vi "upload_data_db.vi"() -> ()   [LabVIEW 2021]
uses:
  <vilib>/Utility/file.llb/Read Delimited Spreadsheet (string).vi
panel:
  in  "function name 2":string="debugprint"
  out "Debug String Out":string="postgres"
  in  "Debug":bool
  out "String Out":string="Upload Success"
  in  "Data cluster":T1={"type"="proto", " geometry"="full", "resolution"="LD", "baselayer"="BA_123", "toplayer"="SI_789", "pos"="1", "region"="1", "asstray"="1", "comptray"="1", "put"="1", "date"="2024-04-02", "timestart"="1:12:12.442", "timeend"="1:23:45.244", "operator"="cmuperson", "tape"="some", "glue"="some"}
  out "Execution Time py":dbl=14.0
  in  "Python version":string="3.7.0"
  in  "stop":bool
  in  "Run Python":bool
  in  "function name":string="assembly_data"
  in  "module path":path=path "../../../Main VIs/python_db/postgres_tools.py"
  out "error out":errorcluster
  in  "error in (no error)":errorcluster
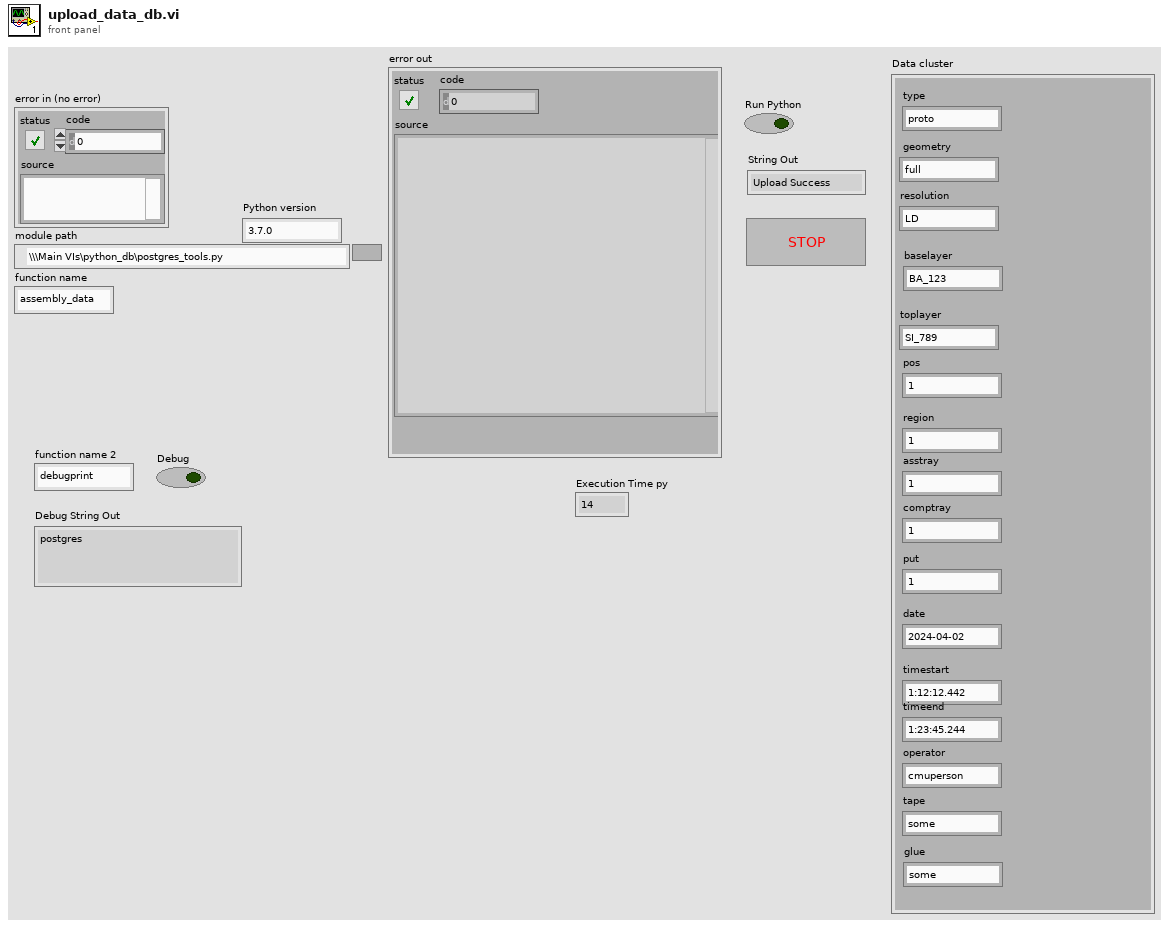
[diagram p1: front panel]
types:
  T1 = cluster{"type":string, " geometry":string, "resolution":string, "baselayer":string, "toplayer":string, "pos":string, "region":string, "asstray":string, "comptray":string, "put":string, "date":string, "timestart":string, "timeend":string, "operator":string, "tape":string, "glue":string}
  T2 = typedef "File Paths.ctl" = cluster{"Glue Pattern Folder":path, "Carrier Tray Folder":path, "Pick Up Tool Fixture Folder":path, "Components Folder":path, "Bellows Tool Offset.txt":path, "Pick Up Tool Offset.txt":path, "Dispense Tip Offset.txt":path, "Log Files":path, "Gantry Assembly Map.txt":path, "Syringe and offset map.txt":path, "Python DB Conn":path}
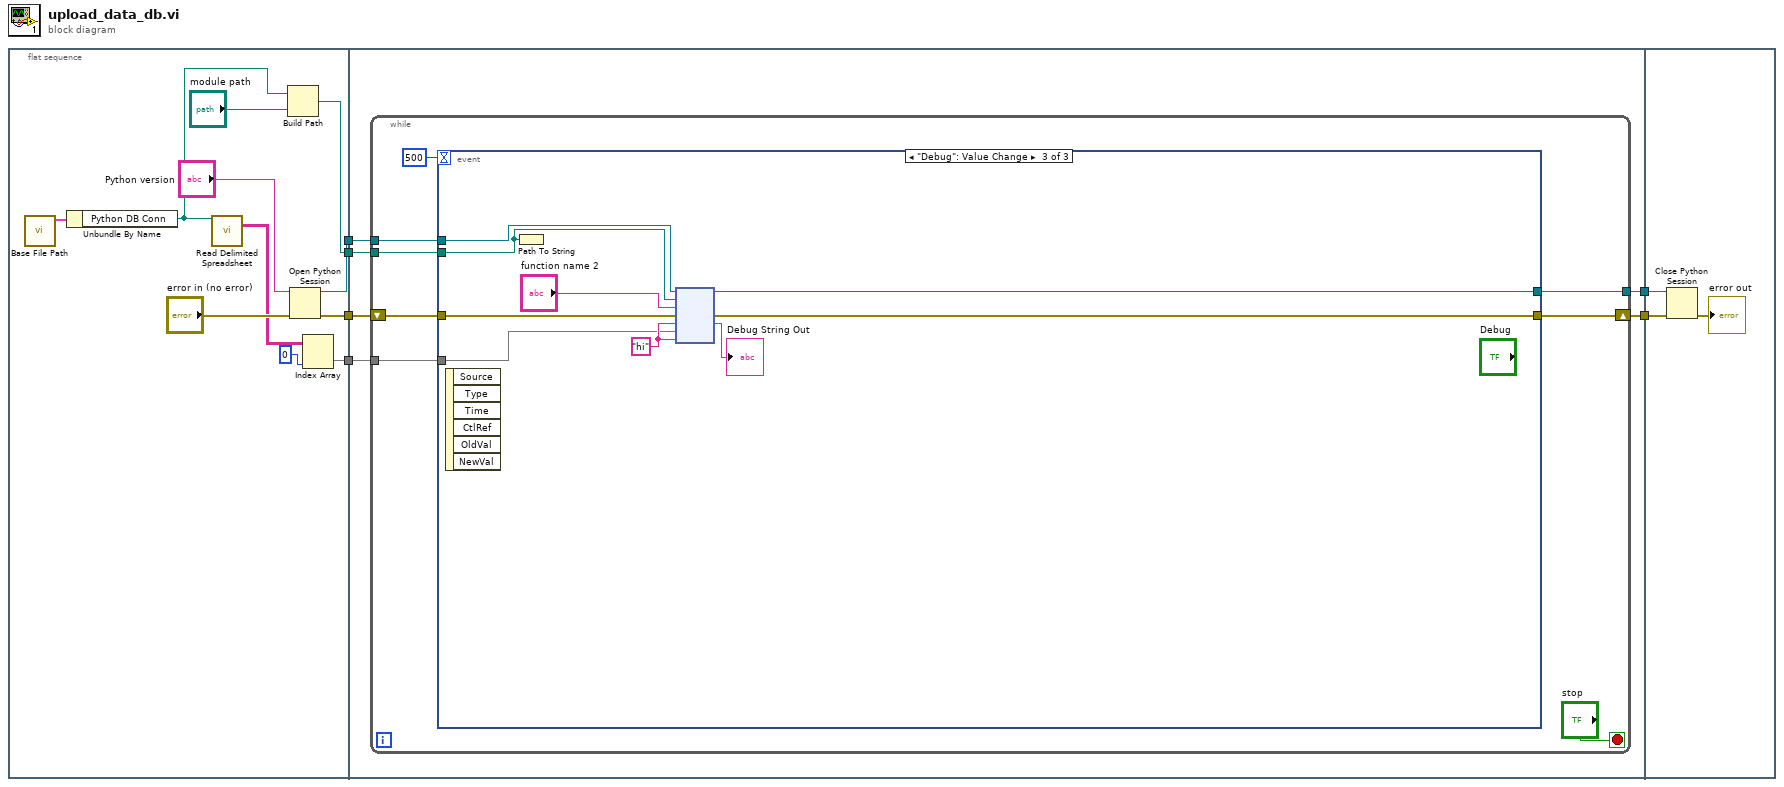
[diagram p0: block diagram]
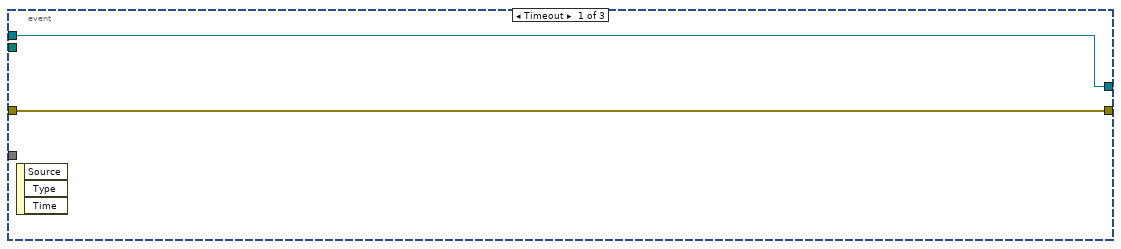
[diagram p2: hidden frame]
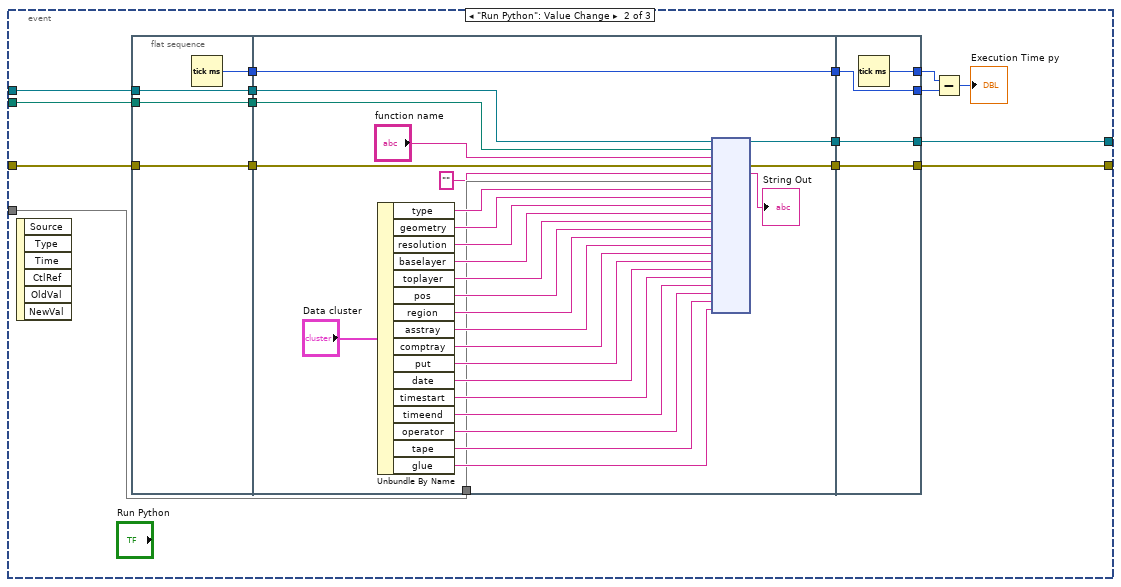
[diagram p3: hidden frame]
diagram:
  n1 = flat-sequence {
    tunnel: [w16] -> w4
    tunnel: [w17] -> w3
    tunnel: [w12] -> w2
    tunnel: [w7] -> w1
    tunnel: [w22] -> w6
    tunnel: [w21] -> w5
    tunnel: w4 -> [w23]
    tunnel: w3 -> [w20]
    tunnel: w2 -> [w19]
    tunnel: w1 -> [w18]
    tunnel: w6 -> [w95]
    tunnel: w5 -> [w96]
    frame #0 {
      n2 = call "Base File Path.vi"() -> ("Paths Out"=w13:T2)  [unwired: 11 in]
      n3 = Unbundle By Name(w13) -> ("Python DB Conn"=w10:path)
      n4 = call-poly <vilib>:"Read Delimited Spreadsheet.vi"("file path (dialog if empty)"=w10) -> ("all rows"=w9:string[][])  [unwired: 9 in, 5 out]
      n5 = Build Path(base path=w10, name or relative path="module path") -> (appended path=w12:path)
      n6 = Open Python Session(python version="Python version", 3:"error in (no error)") -> (session out=w17:refnum<k35>, error out=w16:errorcluster)  [unwired: 1 in]
      n7 = Index Array(array=w9, index (col)=0 ("disabled index (col)")) -> (element=w7:string[])  [unwired: 1 in]
    }
    frame #1 {
      n8 = while {
        shift-right: [w29] -> w22
        shift-left: w23 -> [w30]
        tunnel: w20 -> [w27]
        tunnel: [w28] -> w21
        tunnel: w19 -> [w25]
        tunnel: w18 -> [w24]
        stop <- "stop" stop-if-true
        n9 = event shown="[2] \"Debug\": Value Change" {
          selector: _ -> [_ _ _]
          dyn-events: _ -> [_ _ _]
          timeout: 500 -> [_ _ _]
          tunnel: [w33 w41 w92] -> w29
          tunnel: w30 -> [w33 w44 w93]
          tunnel: [w32 w39 w91] -> w28
          tunnel: w27 -> [w32 w38 w90]
          tunnel: w25 -> [_ w36 w88]
          tunnel: w24 -> [_ w34 w85]
          event Timeout {
            n10 = event-data() -> ()  [unwired: 1 in, 3 out]
          }
          event "Run Python": Value Change {
            n11 = event-data() -> ()  [unwired: 1 in, 6 out]
            n12 = flat-sequence {
              tunnel: [w53] -> w45
              tunnel: w44 -> [w52]
              tunnel: [w52] -> w43
              tunnel: w38 -> [w51]
              tunnel: [w51] -> w37
              tunnel: w36 -> [w50]
              tunnel: [w50] -> w35
              tunnel: [w79] -> w46
              tunnel: w45 -> [w79]
              tunnel: w43 -> [w78]
              tunnel: [w77] -> w42
              tunnel: [w76] -> w40
              tunnel: w37 -> [w75]
              tunnel: w35 -> [w73]
              tunnel: w34 -> [w56]
              tunnel: [w84] -> w48
              tunnel: [w83] -> w47
              tunnel: w46 -> [w83]
              tunnel: w42 -> [w82]
              tunnel: [w82] -> w41
              tunnel: [w81] -> w39
              tunnel: w40 -> [w81]
              frame #0 {
                n13 = Tick Count (ms)() -> (millisecond timer value=w53:u32)
              }
              frame #1 {
                n14 = Unbundle By Name("Data cluster") -> ("type"=w72:string, "geometry"=w71:string, "resolution"=w70:string, "baselayer"=w60:string, "toplayer"=w59:string, "pos"=w58:string, "region"=w57:string, "asstray"=w61:string, "comptray"=w62:string, "put"=w63:string, "date"=w64:string, "timestart"=w65:string, "timeend"=w66:string, "operator"=w67:string, "tape"=w68:string, "glue"=w69:string)
                n15 = node(w75, w73, "function name", w78, "", w56, w72, w71, w70, w60, w59, w58, w57, w61, w62, w63, w64, w65, w66, w67, w68, w69) -> (w76:refnum<k35>, w77:errorcluster, →"String Out":string)  [unwired: 17 in, 2 out]
              }
              frame #2 {
                n16 = Tick Count (ms)() -> (millisecond timer value=w84:u32)
              }
            }
            n17 = Subtract(x=w48, y=w47) -> (x-y=→"Execution Time py":u32)
          }
          event "Debug": Value Change {
            w86 = "hi"
            n18 = event-data() -> ()  [unwired: 1 in, 6 out]
            n19 = Path To String(path=w88) -> ()  [unwired: 1 out]
            n20 = node(w90, w88, "function name 2", w93, w86, w85, w86) -> (w91:refnum<k35>, w92:errorcluster, →"Debug String Out":string)  [unwired: 2 in, 2 out]
          }
        }
      }
    }
    frame #2 {
      n21 = Close Python Session(session in=w96, error in=w95) -> (11:→"error out":errorcluster)
    }
  }
